vi "FTW-Endpoint-Bind-Async.vi"(0 "FTW Endpoint":refnum<class "FTW-Endpoint-Notifier.lvclass">, 5 "Endpoint Address":string, 7 "Requested Identity":string, 11 "error in":errorcluster) -> (4 "FTW Endpoint out":refnum<class "FTW-Endpoint-Notifier.lvclass">, 6 "Actual Endpoint Address":string, 8 "Actual Identity":string, 10 "Incoming Requests":refnum<event-registration>, 15 "error out":errorcluster)   [LabVIEW 2012, in "FTW-Actor.lvlib" / "FTW-Endpoint-Notifier.lvclass"]
uses:
  FTW-Endpoint-Notifier.lvclass
  Message/Request/FTW-Message-IncomingRequest.lvclass
panel:
  # "Inputs"
  # "Outputs"
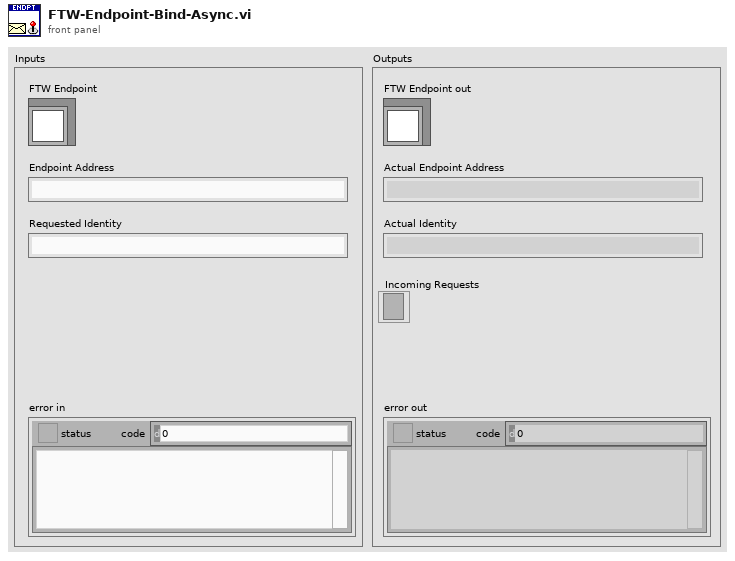
[diagram p1: front panel]
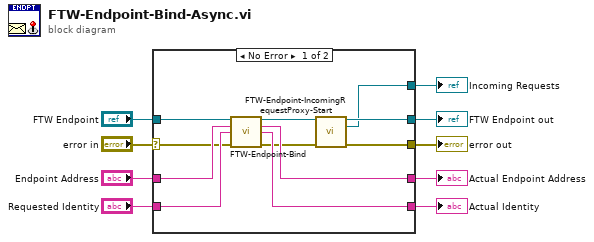
[diagram p0: block diagram]
diagram:
  n1 = case shown="No Error" "error in" {
    selector: "error in" -> [w15 w22]
    tunnel: [w12 w22] -> w9
    tunnel: [w11 w21] -> w7
    tunnel: "FTW Endpoint" -> [w20 w21]
    tunnel: "Requested Identity" -> [w18 _]
    tunnel: "Endpoint Address" -> [w19 _]
    tunnel: [w17 _] -> w3
    tunnel: [w16 _] -> w2
    tunnel: [w10 _] -> w1
    frame No Error {
      n2 = call-dynamic "FTW-Endpoint-Bind.vi"("FTW Endpoint"=w20, "Endpoint Address"=w19, "Requested Identity"=w18, "error in"=w15) -> ("FTW Endpoint out"=w14:refnum<class "FTW-Endpoint-Notifier.lvclass">, "Actual Endpoint Address"=w17:string, "Actual Identity"=w16:string, "error out"=w13:errorcluster)  [unwired: 8 in]
      n3 = call-dynamic "FTW-Endpoint-IncomingRequestProxy-Start.vi"("FTW Endpoint"=w14, "error in"=w13) -> ("FTW Endpoint out"=w11:refnum<class "FTW-Endpoint-Notifier.lvclass">, "Incoming Requests"=w10:refnum<event-registration>, "error out"=w12:errorcluster)  [unwired: 11 in]
    }
    frame Error {
    }
  }
  "error out" <- w9
  "FTW Endpoint out" <- w7
  "Actual Endpoint Address" <- w3
  "Actual Identity" <- w2
  "Incoming Requests" <- w1
